vi "Create Lock.vi"(8 "error in (no error)":errorcluster, 10 "initial lock status (T)":bool=TRUE, 11 "Protected Pointer in":refnum<class "Protected Pointer.lvclass">) -> (0 "error out":errorcluster, 3 "Protected Pointer out":refnum<class "Protected Pointer.lvclass">)   [LabVIEW 2016, in "Memory Manager.lvlib" / "Protected Pointer.lvclass"]
uses:
  Protected Pointer.lvclass
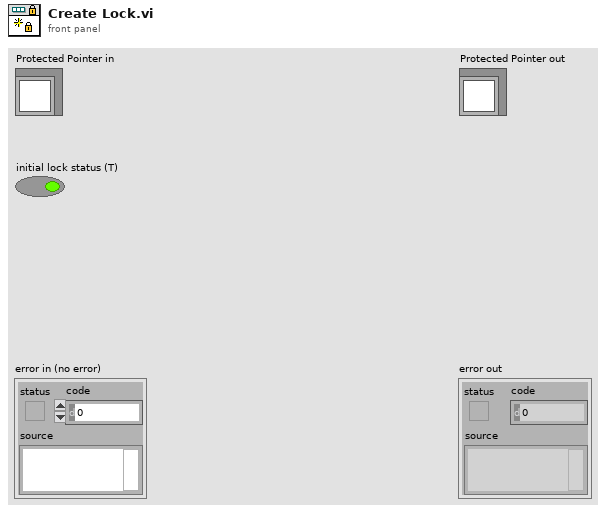
[diagram p1: front panel]
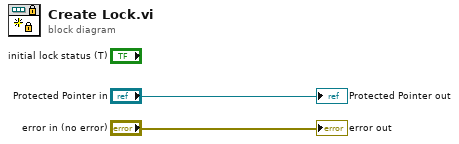
[diagram p0: block diagram]
diagram:
  "error out" <- "error in (no error)"
  "Protected Pointer out" <- "Protected Pointer in"
